vi "Set Plugin Configuration.vi"(8 "error in (no error)":errorcluster, 10 "Plugin Configuration":refnum<class "Configuration.lvclass">, 11 "Component Configuration in":refnum<class "Component Configuration.lvclass">) -> (0 "error out":errorcluster, 3 "Component Configuration out":refnum<class "Component Configuration.lvclass">)   [LabVIEW 2017, in "DSF Core.lvlib" / "Component Configuration.lvclass"]
uses:
  Component Configuration.lvclass
  Configuration/Configuration.lvclass
  Component Configuration.lvclass/Component Configuration.ctl
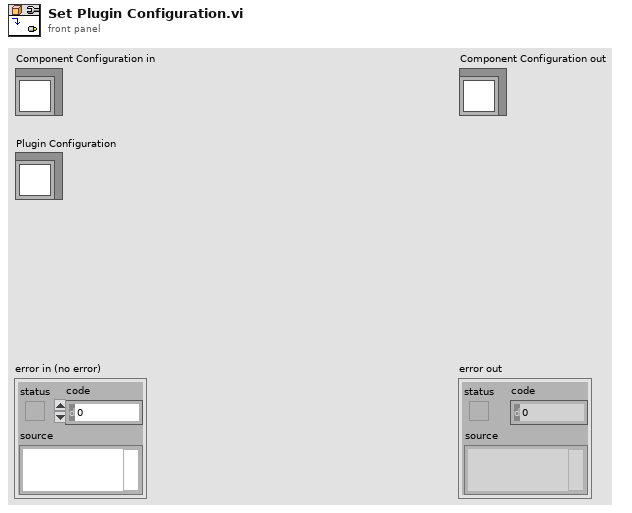
[diagram p1: front panel]
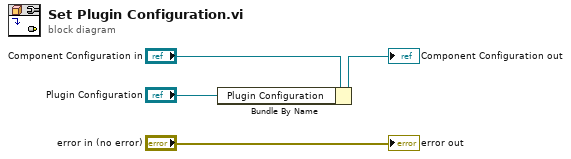
[diagram p0: block diagram]
diagram:
  n1 = Bundle By Name(cluster="Component Configuration in", "Plugin Configuration"="Plugin Configuration") -> (→"Component Configuration out":refnum<class "Component Configuration.lvclass">)
  "error out" <- "error in (no error)"
